vi "Data.vi"(8 "error in (no error)":errorcluster, 11 "Msg in":refnum<class "Msg.lvclass">) -> (0 "error out":errorcluster, 2 "Data":T1 {"Time Stamp" format="%<%x %.3X>T"}, 3 "Msg out":refnum<class "Msg.lvclass">)   [LabVIEW 2023, in "ConstellationCommand.lvlib" / "Msg.lvclass"]
uses:
  Msg.lvclass
  Msg.lvclass/Msg.ctl
  Data.ctl
  ConstellationCommand.lvlib
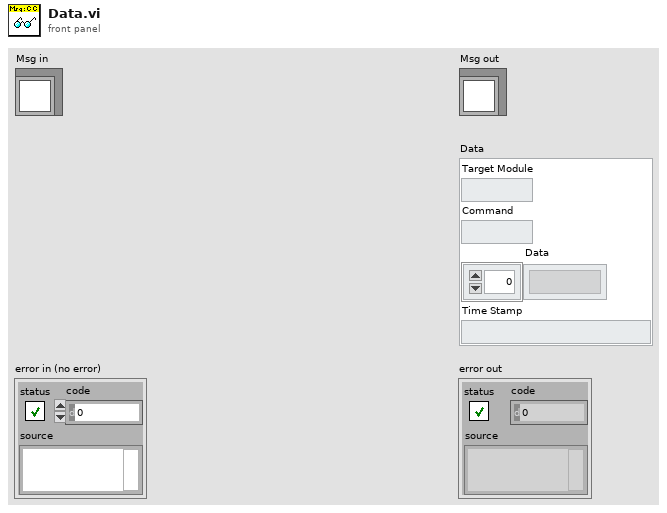
[diagram p1: front panel]
types:
  T1 = typedef "ConstellationCommand.lvlib/Data.ctl" = cluster{"Target Module":string, "Command":string, "Data":string[], "Time Stamp":timestamp}
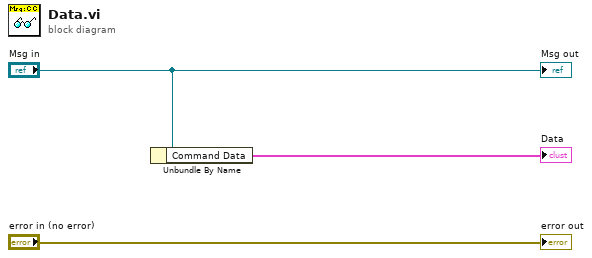
[diagram p0: block diagram]
diagram:
  n1 = Unbundle By Name("Msg in") -> ("Command Data"=→"Data":T1)
  "error out" <- "error in (no error)"
  "Msg out" <- "Msg in"
